vi "16-ParseVersion.vi"(11 "BITS in":bool[](array[boolean])) -> (2 "Version":u32, 3 "BITS out":bool[](array[boolean]))   [LabVIEW 2019, in "16.lvlib"]
uses:
  16.lvlib
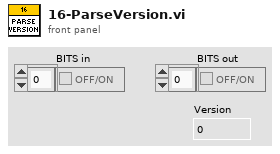
[diagram p1: front panel]
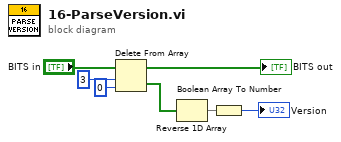
[diagram p0: block diagram]
diagram:
  n1 = Delete From Array(array="BITS in", length=3, index=0) -> (deleted portion=w3:bool[], array with subset deleted=→"BITS out":bool[])
  n2 = Reverse 1D Array(array=w3) -> (reversed array=w6:bool[])
  n3 = Boolean Array To Number(Boolean array=w6) -> (number=→"Version":u32)
